vi "GLOBALS.vi"() -> ()   [LabVIEW 2016]
panel:
  in  "prevz":i16
  in  "prevy":i16
  in  "prevx":i16
  in  "bandwidth":u8
  in  "HPFCutoff":u8
  in  "HPFEnable":u8
  in  "lowPowerEnable":u8
  in  "scale":u16=2000
  in  "_autocalc":bool
  in  "gBiasRaw":u16[](array[numeric])
  in  "gBias":dbl[](array[numeric])
  in  "temperature":u16
  in  "sampleRate":u8=6
  in  "gRes":dbl
  in  "gz":i16
  in  "gy":i16
  in  "gx":i16
  # "float/double"
  # "bool"
  # "uint8"
  # "int16"
  # "uint16"
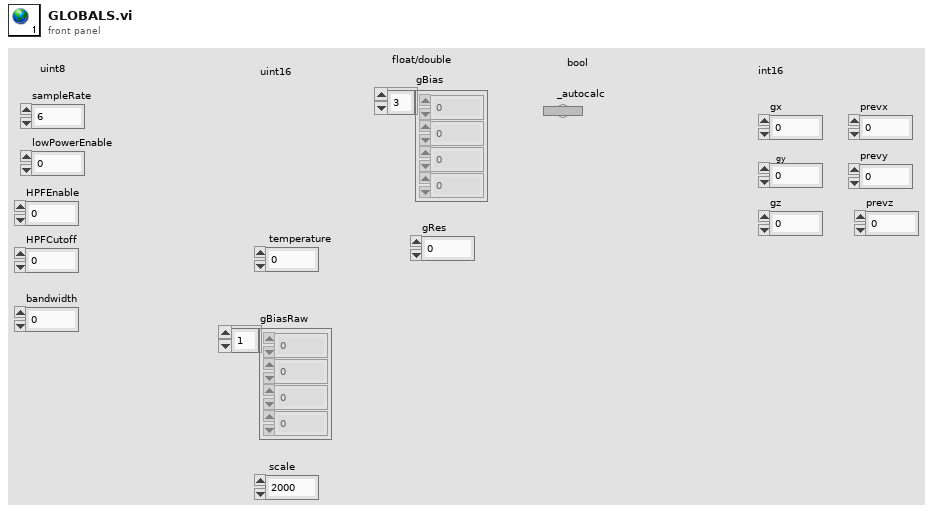
[diagram p1: front panel]
diagram:
